vi "Add Braces String.vi"(1 "String in":string) -> (0 "String out":string)   [LabVIEW 2019, in "Transport.lvclass"]
uses:
  Transport.lvclass
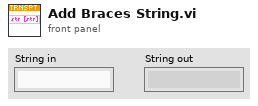
[diagram p1: front panel]
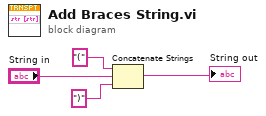
[diagram p0: block diagram]
diagram:
  n1 = Concatenate Strings("(" ("string"), "String in", ")" ("string")) -> (→"String out":string)
